vi "保存数据.vi"(0 "阻变物质":string(combo), 1 "衬底":string(combo), 2 "缓冲区(1)数据未保存":bool, 3 "缓冲区(2)数据未保存":bool) -> (7 "Script":string)   [LabVIEW 2019]
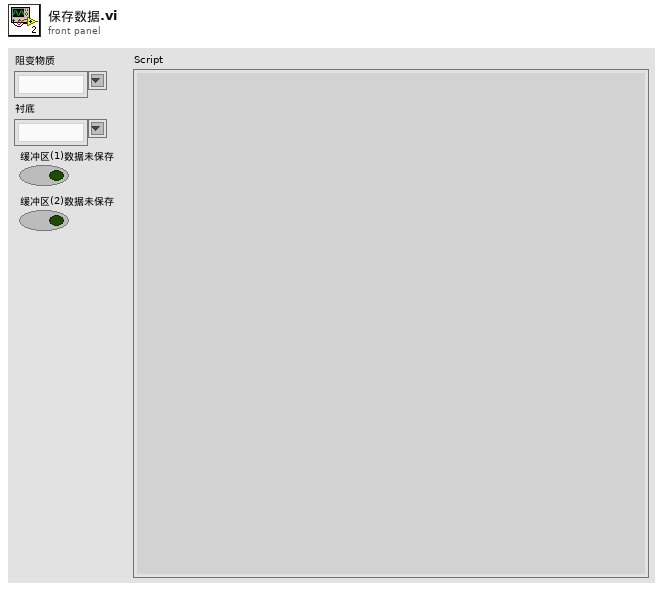
[diagram p1: front panel]
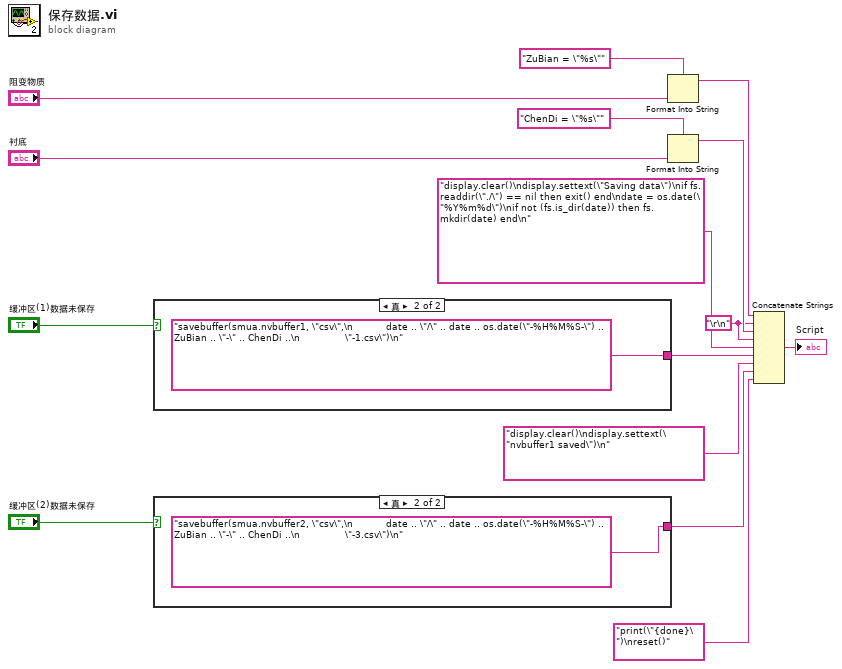
[diagram p0: block diagram]
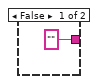
[diagram p2: hidden frame]
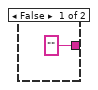
[diagram p3: hidden frame]
diagram:
  w5 = "\r\n"
  n1 = case shown="真" "缓冲区(1)数据未保存" {
    tunnel: ["" "savebuffer(smua.nvbuffer1, \"csv\",\n           date .. \"/\" .. date .. os.date(\"-%H%M%S-\") .. ZuBian .. \"-\" .. ChenDi ..\n               \"-1.csv\")\n"] -> w4
    frame False {
    }
    frame True {
    }
  }
  n2 = case shown="真" "缓冲区(2)数据未保存" {
    tunnel: ["" "savebuffer(smua.nvbuffer2, \"csv\",\n           date .. \"/\" .. date .. os.date(\"-%H%M%S-\") .. ZuBian .. \"-\" .. ChenDi ..\n               \"-3.csv\")\n"] -> w2
    frame False {
    }
    frame True {
    }
  }
  n3 = Format Into String(format string="ZuBian = \"%s\"" ("格式字符串"), "阻变物质") -> (resulting string=w11:string)  [unwired: 2 in, 1 out]
  n4 = Format Into String(format string="ChenDi = \"%s\"" ("格式字符串"), "衬底") -> (resulting string=w10:string)  [unwired: 2 in, 1 out]
  n5 = Concatenate Strings(w11, w5, w10, w5, "display.clear()\ndisplay.settext(\"Saving data\")\nif fs.readdir(\"./\") == nil then exit() end\ndate = os.date(\"%Y%m%d\")\nif not (fs.is_dir(date)) then fs.mkdir(date) end\n", w4, "display.clear()\ndisplay.settext(\"nvbuffer1 saved\")\n", w2, "print(\"{done}\")\nreset()") -> (→"Script":string)
